vi "Timestamp Conversion Array.vi"(9 "timestamps":timestamp[](array[numeric])) -> (2 "timestamps (ns)":i64[](array[numeric]))   [LabVIEW 2026, in "synnax_lib.lvlib"]
uses:
  synnax_lib.lvlib
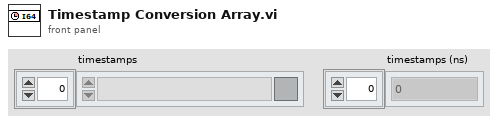
[diagram p1: front panel]
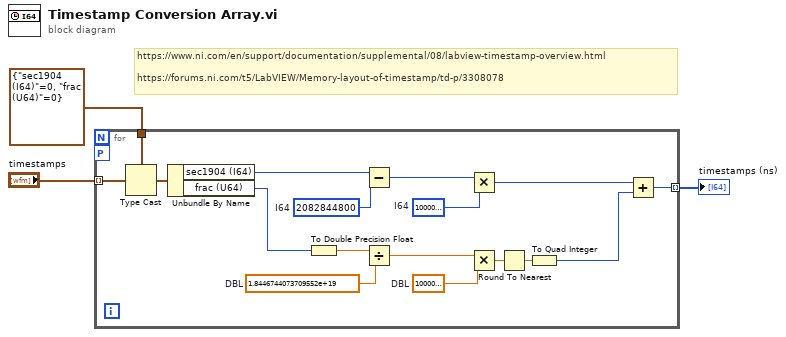
[diagram p0: block diagram]
diagram:
  # "https://www.ni.com/en/support/documentation/supplemental/08/labview-timestamp-overview.html\n\nhttps://forums.ni.com/t5/LabVIEW/Memory-layout-of-timestamp/td-p/3308078"
  n1 = for {
    tunnel: "timestamps" -> [w20] mode=indexing
    workers-P: _ -> [_]
    tunnel: cluster{"sec1904 (I64)":i64, "frac (U64)":u64} {"sec1904 (I64)"=0, "frac (U64)"=0} -> [w19]
    tunnel: [w4] -> w1 mode=indexing
    w9 = 1000000000.0  # DBL
    w11 = 1.8446744073709552e+19  # DBL
    w14 = i64 1000000000  # I64
    w16 = i64 2082844800  # I64
    n2 = Type Cast(type=w19, x=w20) -> (*(type *) &x=w18:cluster{"sec1904 (I64)":i64, "frac (U64)":u64})
    n3 = Unbundle By Name(w18) -> ("sec1904 (I64)"=w17:i64, "frac (U64)"=w13:u64)
    n4 = To Double Precision Float(number=w13) -> (double precision float=w12:dbl)
    n5 = Subtract(x=w17, y=w16) -> (x-y=w15:i64)
    n6 = Divide(x=w12, y=w11) -> (x/y=w10:dbl)
    n7 = Multiply(x=w15, y=w14) -> (x*y=w6:i64)
    n8 = Multiply(x=w10, y=w9) -> (x*y=w8:dbl)
    n9 = Round To Nearest(number=w8) -> (nearest integer value=w7:dbl)
    n10 = To Quad Integer(1:w7) -> (0:w5:i64)
    n11 = Add(x=w6, y=w5) -> (x+y=w4:i64)
  }
  "timestamps (ns)" <- w1
